vi "Save-Load Sys Config.vi"(8 "error in":errorcluster, 9 "System config to save":T1={"XY Stage"={"COM port"="", "XY stage available"=FALSE}, "DAQ FPGA"={"Ref"=refnum, "Target"="RIO0", "Clock Freq (MHz) "=200.0, "input card type"=enum."AC Card", "Samples Wait after Trigger"=5080, "AOD fill"=4900, "StartupDelay"=0, "Slip Cycle (clock cycles)"=600000, "Add Cycle"=TRUE}, "Control system"={"Ethernet opened"=FALSE, "Ethernet Port"=3, "Ctrl FPGA available"=FALSE, "Ctrl FPGA Clock (MHz)"=240.0, "Ctrl system MAC address"="", "Control system.Network adapter name"="", "AOD 1 Amplitude"=0, "AOD 2 Amplitude"=0, "AOD 3 Amplitude"=0, "AOD 4 Amplitude"=0, "Data Time Interval (ns)"=0.0, "T0 (ns)"=0.0, "Ta (ns)"=0.0}, "Encoder"={"IP address"="224.0.1.103", "Port"=7000, "Encoder available"=FALSE, "Wheel radius (cm)"=16.0}, "DAQmx Chan"={"Pockels AO"="", "Hard shutter AO"="", "PMT AOs"="", "Power meter AI"=""}, "Computer MAC address"="", "Cam VidRec"={"DO flag-Video record"="", "DO flag-Trial start"="", "VidRec available"=FALSE}, "Externalise Triggers"=FALSE, "Laser wavelength (nm)"=920.0} {"Laser wavelength (nm)" min=800.0 max=1080.0 step=1.0; "Encoder"."Wheel radius (cm)" format="%#_13g"; "Control system"."Ctrl FPGA Clock (MHz)" min=80.0 max=500.0 step=1.0; "Control system"."Data Time Interval (ns)" min=0.0 max=2048.0 step=1.0; "Control system"."Ta (ns)" min=0.0 max=2048.0 step=1.0; "Control system"."T0 (ns)" min=0.0 max=2048.0 step=1.0; "Control system"."AOD 4 Amplitude" min=0 max=2048 step=1; "Control system"."AOD 3 Amplitude" min=0 max=2048 step=1; "Control system"."AOD 2 Amplitude" min=0 max=2048 step=1; "Control system"."AOD 1 Amplitude" min=0 max=2048 step=1}, 11 "Function":T11=enum."Load from file") -> (0 "error out":errorcluster, 1 "Loaded System config":T1={"XY Stage"={"COM port"="", "XY stage available"=FALSE}, "DAQ FPGA"={"Ref"=refnum, "Target"="RIO0", "Clock Freq (MHz) "=200.0, "input card type"=enum."AC Card", "Samples Wait after Trigger"=5080, "AOD fill"=4900, "StartupDelay"=0, "Slip Cycle (clock cycles)"=600000, "Add Cycle"=TRUE}, "Control system"={"Ethernet opened"=FALSE, "Ethernet Port"=3, "Ctrl FPGA available"=FALSE, "Ctrl FPGA Clock (MHz)"=240.0, "Ctrl system MAC address"="", "Control system.Network adapter name"="", "AOD 1 Amplitude"=0, "AOD 2 Amplitude"=0, "AOD 3 Amplitude"=0, "AOD 4 Amplitude"=0, "Data Time Interval (ns)"=0.0, "T0 (ns)"=0.0, "Ta (ns)"=0.0}, "Encoder"={"IP address"="224.0.1.103", "Port"=7000, "Encoder available"=FALSE, "Wheel radius (cm)"=16.0}, "DAQmx Chan"={"Pockels AO"="", "Hard shutter AO"="", "PMT AOs"="", "Power meter AI"=""}, "Computer MAC address"="", "Cam VidRec"={"DO flag-Video record"="", "DO flag-Trial start"="", "VidRec available"=FALSE}, "Externalise Triggers"=FALSE, "Laser wavelength (nm)"=920.0} {"Laser wavelength (nm)" min=800.0 max=1080.0 step=1.0; "Encoder"."Wheel radius (cm)" format="%#_13g"; "Control system"."Ctrl FPGA Clock (MHz)" min=80.0 max=500.0 step=1.0; "Control system"."Data Time Interval (ns)" min=0.0 max=2048.0 step=1.0; "Control system"."Ta (ns)" min=0.0 max=2048.0 step=1.0; "Control system"."T0 (ns)" min=0.0 max=2048.0 step=1.0; "Control system"."AOD 4 Amplitude" min=0 max=2048 step=1; "Control system"."AOD 3 Amplitude" min=0 max=2048 step=1; "Control system"."AOD 2 Amplitude" min=0 max=2048 step=1; "Control system"."AOD 1 Amplitude" min=0 max=2048 step=1})   [LabVIEW 2013]
uses:
  Typedefs/Sys Configuration.ctl
  Typedefs/XY Stage config cluster.ctl
  Typedefs/DAQ FPGA config cluster.ctl
  RIG-SPECIFIC FILES/FPGA Refs/FPGA Ref.ctl
  <vilib>/userdefined/High Color/nirio_resource_hc.ctl
  Typedefs/FPGA input type AC-DC.ctl
  Typedefs/CTRL system config cluster.ctl
  Typedefs/Encoder config cluster.ctl
  Typedefs/DAQmx physical channels cluster.ctl
  Typedefs/Cam VidRec HW config setup cluster.ctl
  Typedefs/Save-Load enum.ctl
  Typedefs/Which path.ctl
  <vilib>/Utility/config.llb/NI_LVConfig.lvlib
panel:
  # "<--- The \"PMT AOs\" DAQmx string will always contain\n                       2 channels is this format: PXI1Slot4/ao2:3"
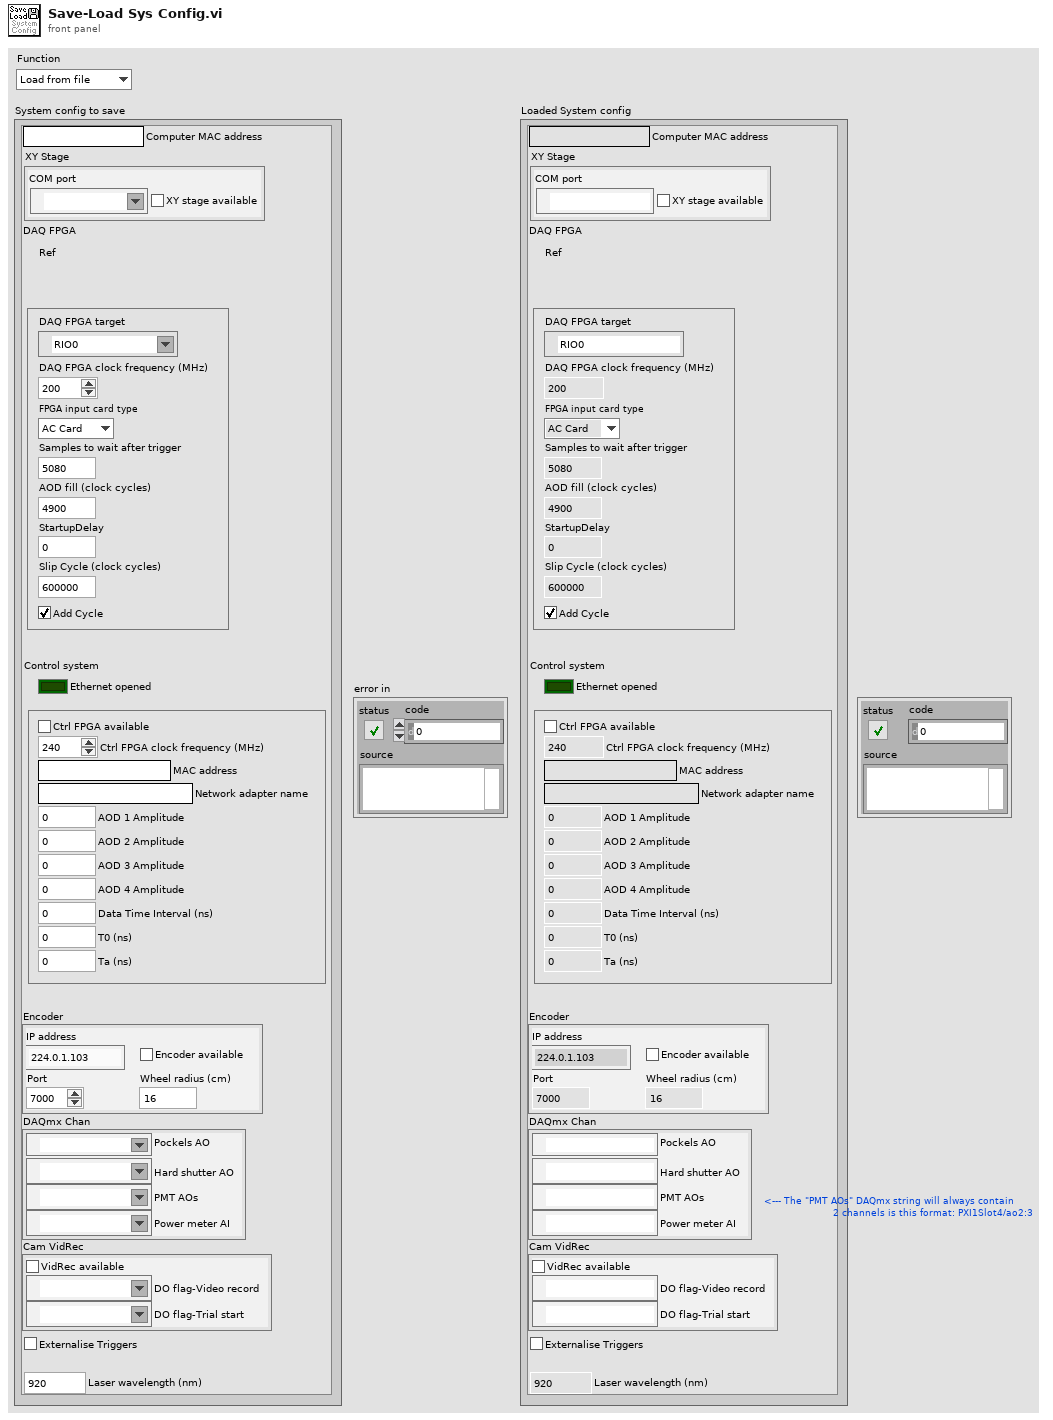
[diagram p1: front panel]
types:
  T1 = typedef "Sys Configuration.ctl" = cluster{"XY Stage":T2, "DAQ FPGA":T3, "Control system":T7, "Encoder":T8, "DAQmx Chan":T9, "Computer MAC address":string, "Cam VidRec":T10, "Externalise Triggers":bool, "Laser wavelength (nm)":dbl}
  T2 = typedef "XY Stage config cluster.ctl" = cluster{"COM port":refnum<visa-resource-name>, "XY stage available":bool}
  T3 = typedef "DAQ FPGA config cluster.ctl" = cluster{"Ref":T4, "Target":T5, "Clock Freq (MHz) ":dbl, "input card type":T6, "Samples Wait after Trigger":u16, "AOD fill":u16, "StartupDelay":i32, "Slip Cycle (clock cycles)":u32, "Add Cycle":bool}
  T4 = typedef "FPGA Ref.ctl" = refnum<k20>
  T5 = typedef "nirio_resource_hc.ctl" = tag
  T6 = typedef "FPGA input type AC-DC.ctl" = enum16{"AC Card", "DC Card"}
  T7 = typedef "CTRL system config cluster.ctl" = cluster{"Ethernet opened":bool, "Ethernet Port":u32, "Ctrl FPGA available":bool, "Ctrl FPGA Clock (MHz)":dbl, "Ctrl system MAC address":string, "Control system.Network adapter name":string, "AOD 1 Amplitude":i16, "AOD 2 Amplitude":i16, "AOD 3 Amplitude":i16, "AOD 4 Amplitude":i16, "Data Time Interval (ns)":dbl, "T0 (ns)":dbl, "Ta (ns)":dbl}
  T8 = typedef "Encoder config cluster.ctl" = cluster{"IP address":string, "Port":u16, "Encoder available":bool, "Wheel radius (cm)":dbl}
  T9 = typedef "DAQmx physical channels cluster.ctl" = cluster{"Pockels AO":tag, "Hard shutter AO":tag, "PMT AOs":tag, "Power meter AI":tag}
  T10 = typedef "Cam VidRec HW config setup cluster.ctl" = cluster{"DO flag-Video record":tag, "DO flag-Trial start":tag, "VidRec available":bool}
  T11 = typedef "Save-Load enum.ctl" = enum16{"Save to file", "Load from file", "Compare from file"}
  T12 = typedef "Which path.ctl" = enum16{"Configuration Files", "Calibration Files", "Images", "Setup.ini", "Loaded User profile.ini", "User's-Previous session.ini", "New user profile.ini", "Selected User profile.ini", "User profiles folder", "Power meter scaling.txt", "FOV Cal.ini"}
  T13 = typedef "NI_LVConfig.lvlib/Config Data RefNum.ctl" = refnum<k1>
  T14 = typedef "Ini file interface (DBL).ctl" = cluster{"key":string, "Save?":bool, "Default":dbl}[]
  T15 = typedef "Ini file interface (String).ctl" = cluster{"key":string, "Save?":bool, "Default":string}[]
  T16 = typedef "Ini file interface (Boolean).ctl" = cluster{"key":string, "Save?":bool, "Default":bool}[]
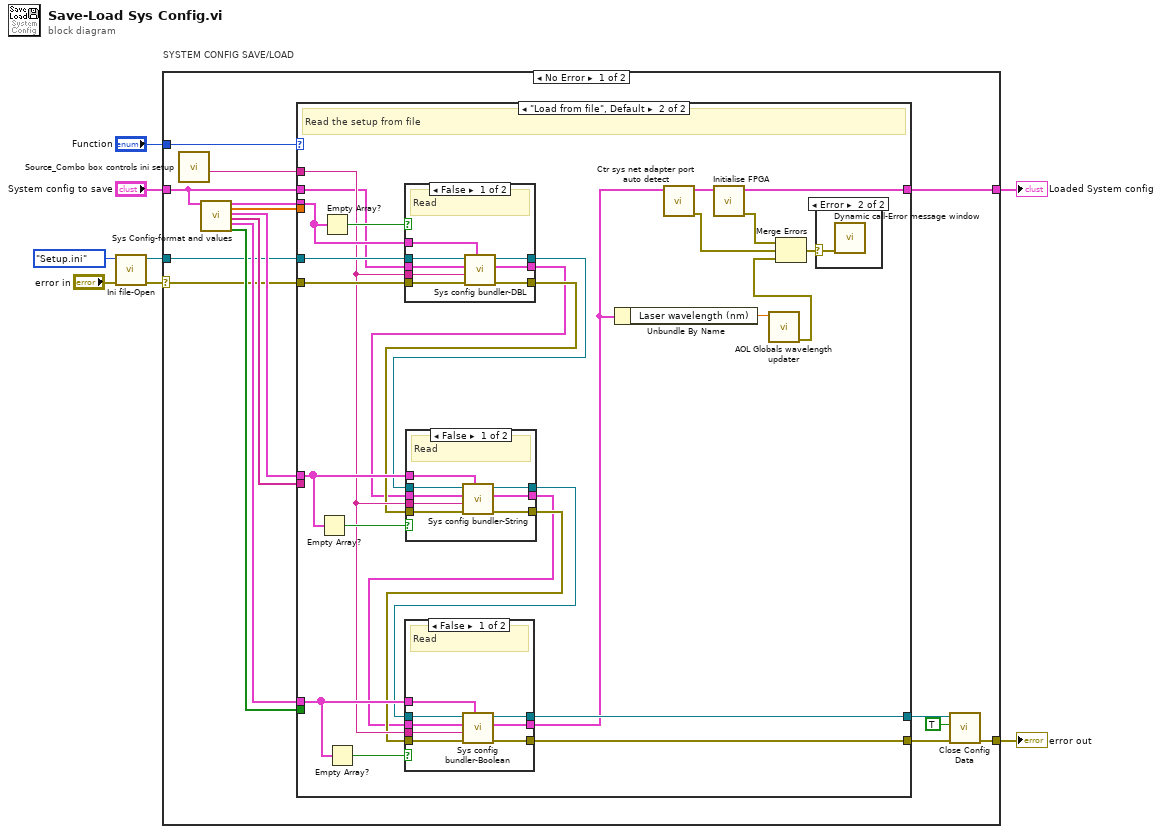
[diagram p0: block diagram]
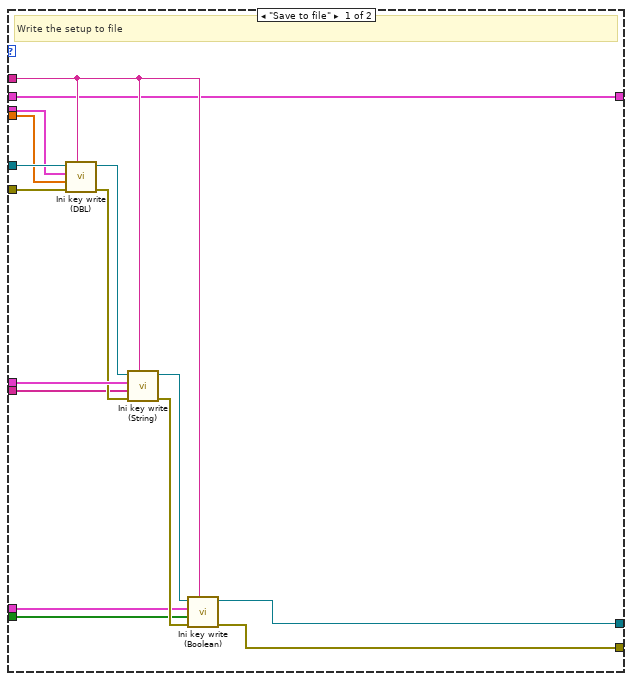
[diagram p2: hidden frame]
diagram:
  n1 = call "Ini file-Open.vi"("Error In"="error in", "Which file?"=Which_path."Setup.ini") -> ("error out"=w4:errorcluster, "User profile ini file ref"=w2:T13)  [unwired: 6 in, 2 out]
  n2 = case "SYSTEM CONFIG SAVE/LOAD" shown="No Error" w4 {
    selector: w4 -> [w13 w102]
    tunnel: [w11 w102] -> w1
    tunnel: "System config to save" -> [w21 w101]
    tunnel: [w22 w101] -> w7
    tunnel: "Function" -> [w14 _]
    tunnel: w2 -> [w12 _]
    frame No Error {
      n3 = call "Source_Combo box controls ini setup.vi"() -> ("Section name"=w9:string)  [unwired: 10 in, 1 out]
      n4 = call "Sys Config-format and values.vi"("System Config"=w21) -> ("Keys setup.DBL"=w20:T14, "Values.DBL"=w19:dbl[], "Keys setup.String"=w18:T15, "Values.Strings"=w17:string[], "Keys setup.Boolean"=w16:T16, "Values.Boolean"=w15:bool[])  [unwired: 13 in]
      n5 = case shown="\"Load from file\", Default" w14 {
        tunnel: [w27 w61] -> w10
        tunnel: [w26 w62] -> w23
        tunnel: w13 -> [w39 w63]
        tunnel: w12 -> [w40 w66]
        tunnel: w9 -> [w29 w56]
        tunnel: w20 -> [w37 w65]
        tunnel: w19 -> [w38 _]
        tunnel: w15 -> [w28 _]
        tunnel: w16 -> [w30 w60]
        tunnel: w17 -> [w33 _]
        tunnel: w18 -> [w36 w57]
        tunnel: [w25 w46] -> w22
        tunnel: w21 -> [w25 w51]
        frame "Save to file" {
          # "Write the setup to file"
          n6 = call "Ini key write (DBL).vi"("Section"=w29, "error in (no error)"=w39, "Values (DBL)"=w38, "Ini file interface"=w37, "Ini file refnum in"=w40) -> ("error out"=w34:errorcluster, "Ini file refnum out"=w35:T13)  [unwired: 5 in]
          n7 = call "Ini key write (String).vi"("Section"=w29, "error in (no error)"=w34, "Values (String)"=w33, "Ini file interface"=w36, "Ini file refnum in"=w35) -> ("error out"=w31:errorcluster, "Ini file refnum out"=w32:T13)  [unwired: 5 in]
          n8 = call "Ini key write (Boolean).vi"("Section"=w29, "error in (no error)"=w31, "Values (Boolean)"=w28, "Ini file interface"=w30, "Ini file refnum in"=w32) -> ("error out"=w27:errorcluster, "Ini file refnum out"=w26:T13)  [unwired: 5 in]
        }
        frame "Load from file", Default {
          # "Read the setup from file"
          n9 = Empty Array?(array=w57) -> (empty?=w58:bool)
          n10 = Empty Array?(array=w65) -> (empty?=w64:bool)
          n11 = Empty Array?(array=w60) -> (empty?=w59:bool)
          n12 = case shown="False" w64 {
            tunnel: w66 -> [w97 w100]
            tunnel: [w96 w100] -> w52
            tunnel: [w95 w99] -> w53
            tunnel: w63 -> [w94 w99]
            tunnel: w56 -> [w92 _]
            tunnel: w65 -> [w93 _]
            tunnel: w51 -> [w91 w98]
            tunnel: [w90 w98] -> w50
            frame False {
              # "Read"
              n13 = call "Sys config bundler-DBL.vi"("Keys setup.DBL"=w93, "error in (no error)"=w94, "Section name"=w92, "System Config to save in"=w91, "Refnum in"=w97) -> ("error out"=w95:errorcluster, "System Config to save out"=w90:T1, "Refnum out"=w96:T13)  [unwired: 4 in]
            }
            frame True {
              # "No parametersof such type"
            }
          }
          n14 = case shown="False" w58 {
            tunnel: [w72 w78] -> w55
            tunnel: [w71 w77] -> w54
            tunnel: w57 -> [w74 _]
            tunnel: w52 -> [w75 w78]
            tunnel: w53 -> [w70 w77]
            tunnel: w56 -> [w73 _]
            tunnel: w50 -> [w69 w76]
            tunnel: [w68 w76] -> w49
            frame False {
              # "Read"
              n15 = call "Sys config bundler-String.vi"("Keys setup.String"=w74, "error in (no error)"=w70, "Section name"=w73, "System Config to save in"=w69, "Refnum in"=w75) -> ("error out"=w71:errorcluster, "System Config to save out"=w68:T1, "Refnum out"=w72:T13)  [unwired: 4 in]
            }
            frame True {
              # "No parametersof such type"
            }
          }
          n16 = case shown="False" w59 {
            tunnel: [w85 w89] -> w62
            tunnel: [w84 w88] -> w61
            tunnel: w60 -> [w81 _]
            tunnel: w55 -> [w86 w89]
            tunnel: w54 -> [w83 w88]
            tunnel: w56 -> [w82 _]
            tunnel: w49 -> [w80 w87]
            tunnel: [w79 w87] -> w43
            frame False {
              # "Read"
              n17 = call "Sys config bundler-Boolean.vi"("Keys setup.Boolean"=w81, "error in (no error)"=w83, "Section name"=w82, "System Config to save in"=w80, "Refnum in"=w86) -> ("error out"=w84:errorcluster, "System Config to save"=w79:T1, "Refnum out"=w85:T13)  [unwired: 4 in]
            }
            frame True {
              # "No parametersof such type"
            }
          }
          n18 = Unbundle By Name(w43) -> ("Laser wavelength (nm)"=w44:dbl)
          n19 = call "Ctr sys net adapter port auto detect.vi"("Sys Config to save in"=w43) -> ("error out"=w42:errorcluster, "Sys Config to save out"=w48:T1)  [unwired: 9 in]
          n20 = call "Initialise FPGA.vi"("Hardware Resources in"=w48) -> ("error out"=w41:errorcluster, "Hardware Resources out"=w46:T1)  [unwired: 9 in]
          n21 = call "AOL Globals wavelength updater.vi"("Laser wavelength (nm)"=w44) -> ("error out"=w45:errorcluster)  [unwired: 10 in]
          n22 = Merge Errors(w41, w42, w45) -> (w47:errorcluster)
          n23 = case shown="Error" w47 {
            selector: w47 -> [_ w67]
            frame No Error {
            }
            frame Error {
              n24 = call "Dynamic call-Error message window.vi"("error in (no error)"=w67) -> ()  [unwired: 10 in, 1 out]
            }
          }
        }
      }
      n25 = call <vilib>:"Close Config Data.vi"("error in (no error)"=w10, "write file if changed (T)"=TRUE ("write configuration file? (F)"), "refnum"=w23) -> ("error out"=w11:errorcluster)  [unwired: 7 in, 1 out]
    }
    frame Error {
    }
  }
  "error out" <- w1
  "Loaded System config" <- w7
